vi "MagnetControl.vi"(8 "error in (no error)":errorcluster, 11 "VISA resource name":refnum<visa-resource-name>="ipsetherB") -> (0 "error out":errorcluster)   [LabVIEW 2017]
uses:
  controls/iPSreadCtrl.ctl
  controls/iPSsetCtrl.ctl
panel:
  out "Monitor":T1(graph)
  in  "Target Field, T":dbl min=-18.0 max=18.0 step=0.01
  in  "iPSSetCtrl":T2
  in  "Field Rate, T/min":dbl min=0.0 max=0.2 step=0.0001
  out "Magnet Readings":T3={"Signals"=["Output Field (T)", "Magnet Field (T)", "Switch Heater Temp (K)", "Field Rate (T/min)", "Magnet Temp (T)"], "Magnet Readings"=[0.0, -1.2307692307692308e-05, 291.0928, 0.1, 290.5584]}
  in  "iPSreadCtrl":T4=enum."Switch Heater Temp"
  in  "Set":bool
  in  "Refresh Time (ms)":i32=100
  in  "Quit":bool
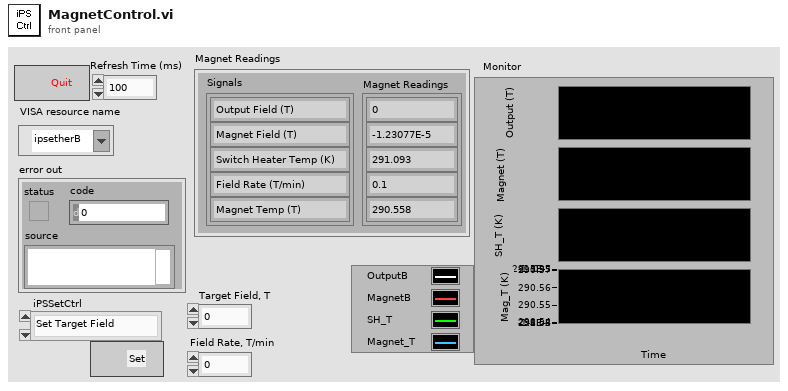
[diagram p1: front panel]
types:
  T1 = cluster{"number":dbl, "number":dbl, "number":dbl, "number":dbl}
  T2 = typedef "iPSsetCtrl.ctl" = enum16{"Set Target Field", "Set Target Field Rate", "Switch Heater ON", "Switch Heater OFF", "Go to Field", "Go to Zero", "Hold"}
  T3 = cluster{"Signals":string[], "Magnet Readings":dbl[]}
  T4 = typedef "iPSreadCtrl.ctl" = enum16{"OutputField", "MagnetField", "Switch Heater Temp", "Field Rate", "Magnet Temp"}
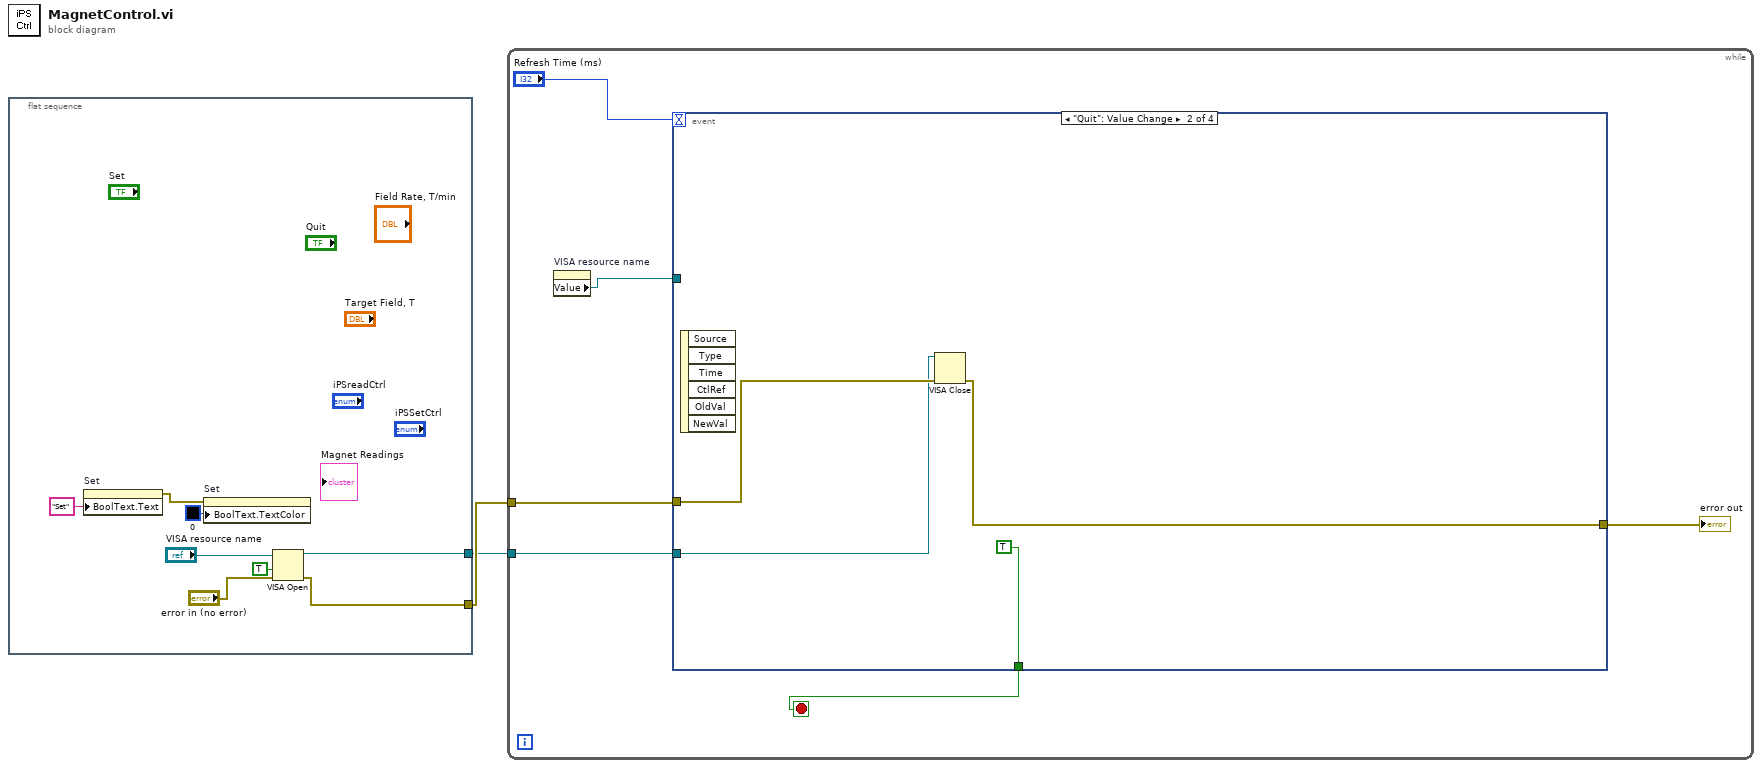
[diagram p0: block diagram]
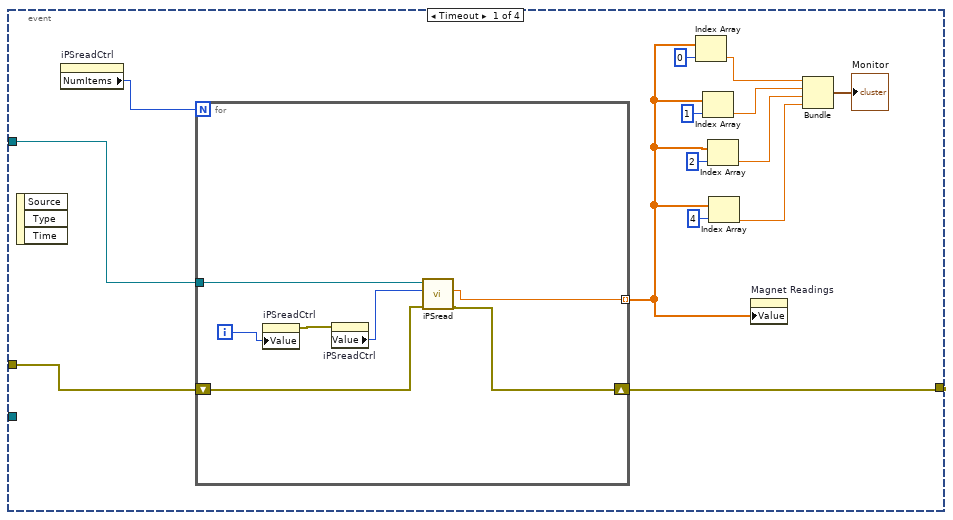
[diagram p2: hidden frame]
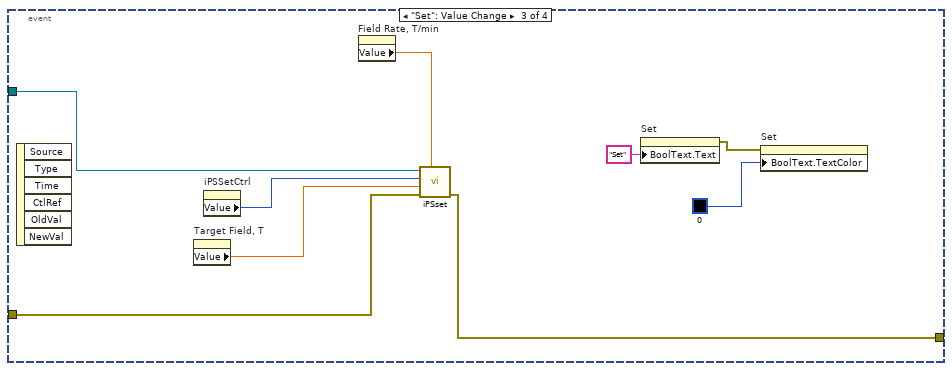
[diagram p3: hidden frame]
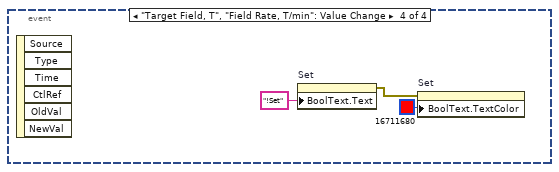
[diagram p4: hidden frame]
diagram:
  n1 = flat-sequence {
    tunnel: [w5] -> w2
    tunnel: [w3] -> w1
    frame #0 {
      n2 = property on="Set" class="Bool (strict)"("BoolText.Text"="Set" ("Boolean Text.Text")) -> (error out=w10:errorcluster)  [unwired: 2 in, 1 out]
      n3 = property on="Set" class="Bool (strict)"(error in=w10, "BoolText.TextColor"=u32 0 ("Boolean Text.Colors:BG Color")) -> ()  [unwired: 1 in, 2 out]
      n4 = VISA Open(duplicate session (F)=TRUE, error in (no error)="error in (no error)", VISA resource name="VISA resource name") -> (VISA resource name=w3:refnum<visa-resource-name>, error out=w5:errorcluster)  [unwired: 2 in]
    }
  }
  n5 = while {
    tunnel: w2 -> [w15]
    tunnel: w1 -> [w12]
    stop <- w14 stop-if-true
    n6 = property on="VISA resource name" class="VISAName"() -> ("Value"=w11:refnum<visa-resource-name>)  [unwired: 2 in, 2 out]
    n7 = event shown="[1] \"Quit\": Value Change" {
      selector: _ -> [_ _ _ _]
      dyn-events: _ -> [_ _ _ _]
      timeout: "Refresh Time (ms)" -> [_ _ _ _]
      tunnel: w15 -> [w30 w40 w44 _]
      tunnel: [w29 w39 w43 _] -> w13
      tunnel: [_ TRUE _ _] -> w14
      tunnel: w12 -> [_ w38 _ _]
      tunnel: w11 -> [w17 _ w42 _]
      event Timeout {
        n8 = event-data() -> ()  [unwired: 1 in, 3 out]
        n9 = property on="iPSreadCtrl" class="Enum (strict)"() -> ("NumItems"=w28:u32)  [unwired: 2 in, 2 out]
        n10 = for {
          N: w28 -> [_]
          shift-right: [w36] -> w29
          shift-left: w30 -> [w37]
          tunnel: [w35] -> w19 mode=indexing
          tunnel: w17 -> [w31]
          i -> [w34]
          n11 = property on="iPSreadCtrl" class="Enum (strict)"("Value"=w34) -> (error out=w33:errorcluster)  [unwired: 2 in, 1 out]
          n12 = property on="iPSreadCtrl" class="Enum (strict)"(error in=w33) -> ("Value"=w32:T4)  [unwired: 1 in, 2 out]
          n13 = call "iPSread.vi"("error in (no error)"=w37, "iPSreadCtrl"=w32, "VISA resource name"=w31) -> ("error out"=w36:errorcluster, "number"=w35:dbl)  [unwired: 5 in, 2 out]
        }
        n14 = Index Array(array=w19, index=0) -> (element=w24:dbl)
        n15 = Index Array(array=w19, index=1) -> (element=w22:dbl)
        n16 = Index Array(array=w19, index=2) -> (element=w18:dbl)
        n17 = Index Array(array=w19, index=4) -> (element=w21:dbl)
        n18 = property on="Magnet Readings" class="Arr (strict)"("Value"=w19) -> ()  [unwired: 2 in, 2 out]
        n19 = Bundle("number"=w24, "number"=w22, "number"=w18, "number"=w21) -> (→"Monitor":T1)  [unwired: 1 in]
      }
      event "Quit": Value Change {
        n20 = event-data() -> ()  [unwired: 1 in, 6 out]
        n21 = VISA Close(VISA resource name=w38, error in (no error)=w40) -> (error out=w39:errorcluster)
      }
      event "Set": Value Change {
        n22 = event-data() -> ()  [unwired: 1 in, 6 out]
        n23 = property on="Target Field, T" class="DigNum (strict)"() -> ("Value"=w45:dbl)  [unwired: 2 in, 2 out]
        n24 = property on="iPSSetCtrl" class="Enum (strict)"() -> ("Value"=w46:T2)  [unwired: 2 in, 2 out]
        n25 = property on="Field Rate, T/min" class="DigNum (strict)"() -> ("Value"=w47:dbl)  [unwired: 2 in, 2 out]
        n26 = call "iPSset.vi"("Field Rate, T/min"=w47, "error in (no error)"=w44, "Target Field, T"=w45, "iPSSetCtrl"=w46, "VISA resource name"=w42) -> ("error out"=w43:errorcluster)  [unwired: 3 in, 3 out]
        n27 = property on="Set" class="Bool (strict)"("BoolText.Text"="Set" ("Boolean Text.Text")) -> (error out=w48:errorcluster)  [unwired: 2 in, 1 out]
        n28 = property on="Set" class="Bool (strict)"(error in=w48, "BoolText.TextColor"=u32 0 ("Boolean Text.Colors:BG Color")) -> ()  [unwired: 1 in, 2 out]
      }
      event "Target Field, T", "Field Rate, T/min": Value Change {
        n29 = event-data() -> ()  [unwired: 1 in, 6 out]
        n30 = property on="Set" class="Bool (strict)"("BoolText.Text"="!Set" ("Boolean Text.Text")) -> (error out=w52:errorcluster)  [unwired: 2 in, 1 out]
        n31 = property on="Set" class="Bool (strict)"(error in=w52, "BoolText.TextColor"=u32 16711680 ("Boolean Text.Colors:BG Color")) -> ()  [unwired: 1 in, 2 out]
      }
    }
    "error out" <- w13
  }
